vi "CAMERA_wait_for_task_DONE.vi"(1 "error in":errorcluster) -> (0 "error out":errorcluster)   [LabVIEW 2015]
uses:
  <vilib>/Utility/error.llb/DialogType.ctl
  GLOBAL/Global_CAMERA.vi
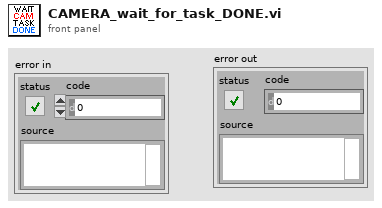
[diagram p1: front panel]
types:
  T1 = typedef "DialogType.ctl" = u16
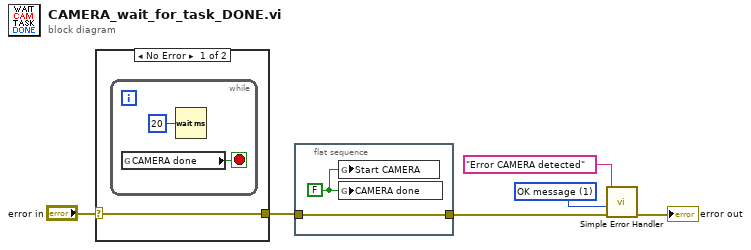
[diagram p0: block diagram]
diagram:
  w4 = T1 1 items=["no dialog", "OK message", "continue or stop message", "OK message + warnings", "continue/stop + warnings"] ("type of dialog (OK msg:1)")
  n1 = case shown="No Error" "error in" {
    selector: "error in" -> [w7 w10]
    tunnel: [w7 w10] -> w1
    frame No Error {
      n2 = while {
        stop <- w9 stop-if-true
        n3 = global read "Global_CAMERA.vi" "CAMERA done"() -> (w9:bool)
        n4 = Wait (ms)(milliseconds to wait=u32 20) -> ()  [unwired: 1 out]
      }
    }
    frame Error {
    }
  }
  n5 = flat-sequence {
    tunnel: [w11] -> w6
    tunnel: w1 -> [w11]
    frame #0 {
      w12 = FALSE ("ANDOR done")
      n6 = global write "Global_CAMERA.vi" "Start CAMERA"(w12) -> ()
      n7 = global write "Global_CAMERA.vi" "CAMERA done"(w12) -> ()
    }
  }
  n8 = call <vilib>:"Simple Error Handler.vi"("error source (\" \")"="Error CAMERA detected" ("error source (\" \")"), "type of dialog (OK msg:1)"=w4, "error in (no error)"=w6) -> ("error out"=→"error out":errorcluster)  [unwired: 2 in, 4 out]
